vi "Loading Screen.vi"() -> ()   [LabVIEW 2014]
uses:
  <vilib>/Utility/miscctls.llb/LVPointTypeDef.ctl
  Stop Button/SubVI/Get Stop Button Status.vi
panel:
  in  "Activate?":bool
  in  "State":T1(ring)=enum."Standard"
  out "error out":errorcluster
  in  "Error In":errorcluster
  out "Message":string
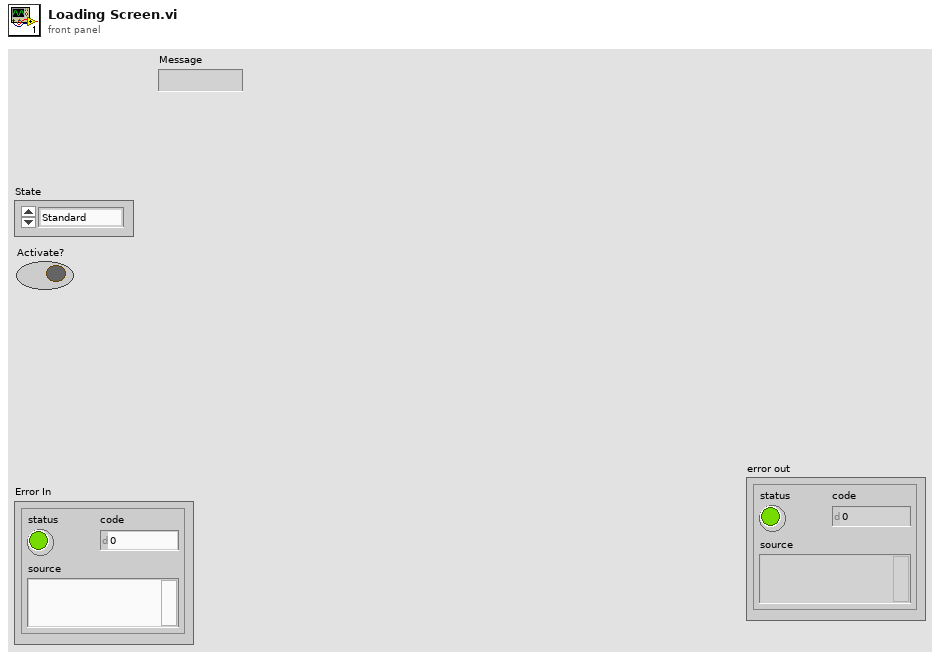
[diagram p1: front panel]
types:
  T1 = enum32{"Invalid", "Standard", "Closed", "Hidden", "Minimized", "Maximized"}
  T2 = typedef "LVPointTypeDef.ctl" = cluster{"Horizontal":i16, "Vertical":i16}
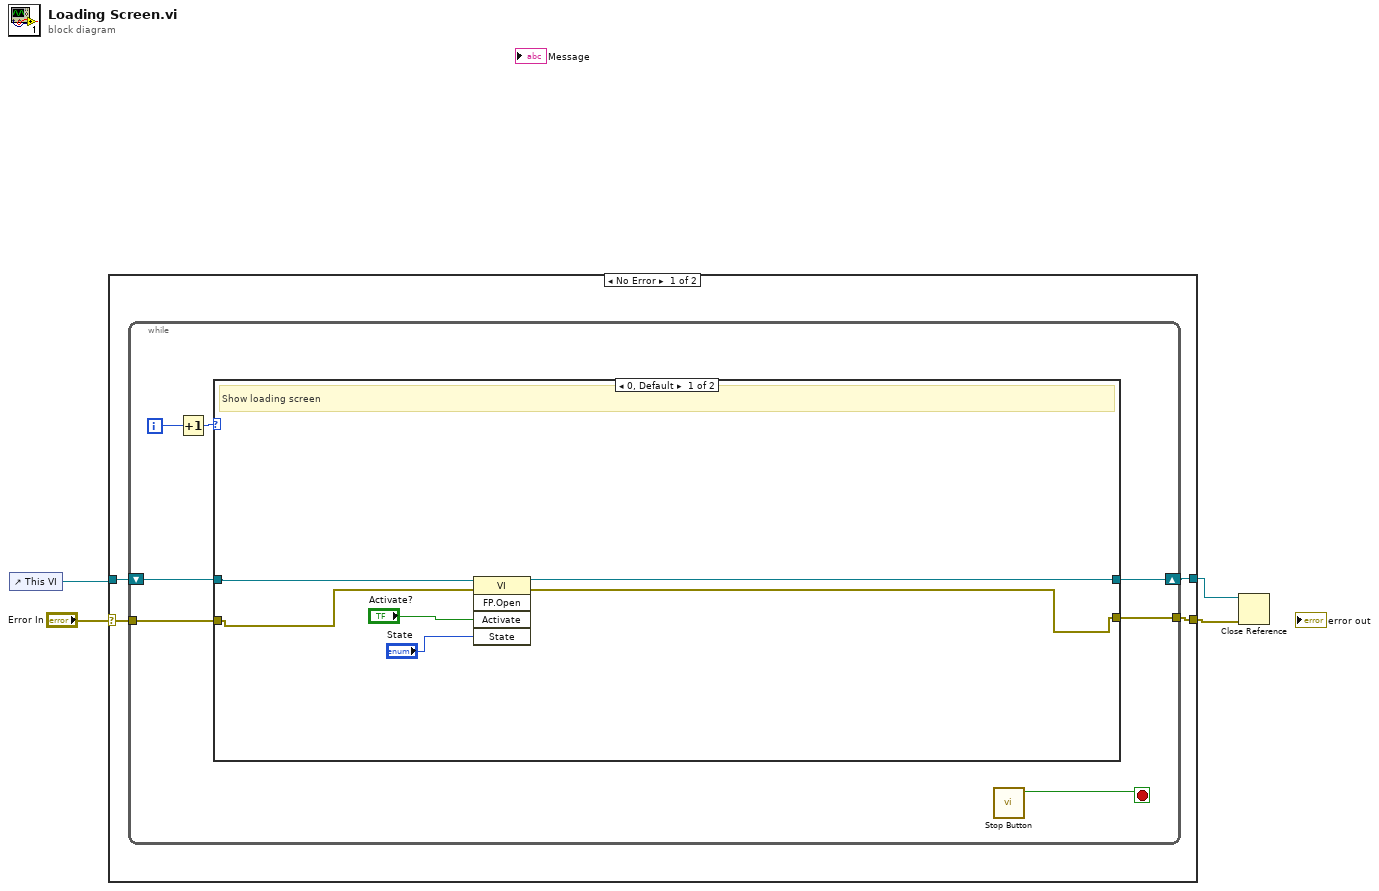
[diagram p0: block diagram]
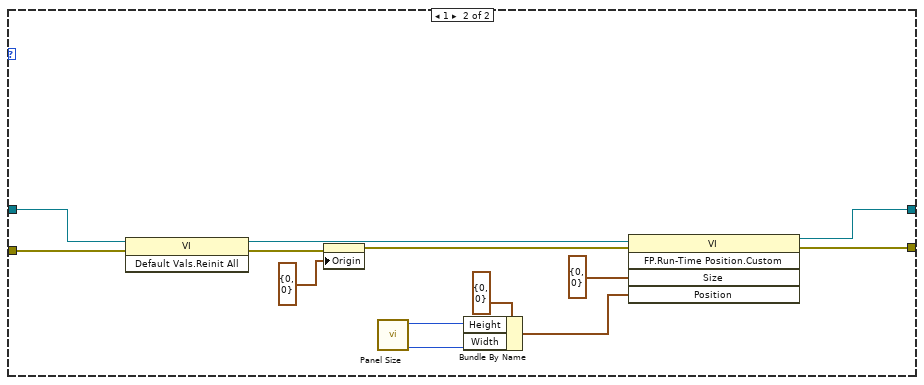
[diagram p2: hidden frame]
diagram:
  n1 = control-ref of="This VI"() -> (w3:refnum<vi>)
  n2 = case shown="No Error" "Error In" {
    selector: "Error In" -> [w7 w37]
    tunnel: [w8 w37] -> w2
    tunnel: w3 -> [w6 w36]
    tunnel: [w5 w36] -> w1
    frame No Error {
      n3 = while {
        tunnel: w7 -> [w13]
        tunnel: [w12] -> w8
        shift-right: [w9] -> w5
        shift-left: w6 -> [w10]
        i -> [w15]
        stop <- w11 stop-if-true
        n4 = Increment(x=w15) -> (x+1=w14:i32)
        n5 = case shown="0, Default" w14 {
          tunnel: w13 -> [w20 w31]
          tunnel: [w17 w23] -> w12
          tunnel: w10 -> [w21 w25]
          tunnel: [w16 w24] -> w9
          frame 0, Default {
            # "Show loading screen"
            n6 = invoke class="VI" method="FP.Open"(reference=w21, error in=w20, "Activate"="Activate?", "State"="State") -> (reference out=w16:refnum<vi>, error out=w17:errorcluster)  [unwired: 1 in, 3 out]
            n7 = Wait (ms)(milliseconds to wait=u32 100) -> ()  [unwired: 1 out]
          }
          frame 1 {
            n8 = invoke class="VI" method="Default Vals.Reinit All"(reference=w25, error in=w31) -> (reference out=w35:refnum<vi>, error out=w34:errorcluster)  [unwired: 1 in, 1 out]
            n9 = property on="Pane" class="Pane"(error in=w34, "Origin"=T2 {"Horizontal"=0, "Vertical"=0}) -> (error out=w33:errorcluster)  [unwired: 1 in, 1 out]
            n10 = call "Panel Size.vi"() -> ("Width In Pixels"=w27:i32, "Height In pixels"=w28:i32)  [unwired: 10 in]
            n11 = Bundle By Name(cluster=cluster{"Height":i16, "Width":i16} {"Height"=0, "Width"=0} ("Size"), "Height"=w28, "Width"=w27) -> (w26:cluster{"Height":i16, "Width":i16})
            n12 = invoke class="VI" method="FP.Run-Time Position.Custom"(reference=w35, error in=w33, "Size"=cluster{"Top":i16, "Left":i16} {"Top"=0, "Left"=0} ("Position"), "Position"=w26) -> (reference out=w24:refnum<vi>, error out=w23:errorcluster)  [unwired: 1 in, 3 out]
          }
        }
        n13 = call-poly "Stop Button.vi"() -> ("Stop ButtonOut"=w11:bool)  [unwired: 10 in, 1 out]
      }
    }
    frame Error {
    }
  }
  n14 = Close Reference(reference=w1, error in (no error)=w2) -> ()  [unwired: 1 out]
